vi "main.vi"() -> ()   [LabVIEW 2025]
uses:
  Module Main Cases.ctl
  71319344-41ff-4242-989e-c571bc358f37.vi
  <vilib>/Utility/error.llb/Clear Errors.vi
  <extravilib>/ChannelInstances/Event Messenger-c(str,var)/Instantiate.vi
  <extravilib>/ChannelInstances/Event Messenger-c(str,var)/))Channel.vi
  Channel Messages/9242 error converting cmd string to case enum--error.vi
  Channel Messages/Bundle Module Message/Bundle Module Message.xnode
  Module2/Module 2.lvlib
  Common-LabVIEW-Helpers/Source/Common Helpers.lvlib
  <extravilib>/ChannelInstances/Event Messenger-c(str,var).lvlib
panel:
  out "Sum Result":dbl
  in  "Sum":bool
  in  "Summand B":dbl
  in  "Summand A":dbl
  out "last ack data":cluster{"ident":string, "error":errorcluster}
  in  "module_interface":map{string, variant}(c390)={"Last Ack"=variant(cluster{"ident":string, "error":errorcluster} {"ident"="", "error"={"status"=FALSE, "code"=0, "source"=""}}), "Sum Result"=variant(dbl 0.0)}
  in  "Show Module2":bool
  in  "Show Module1":bool
  in  "Process Stop Button":bool
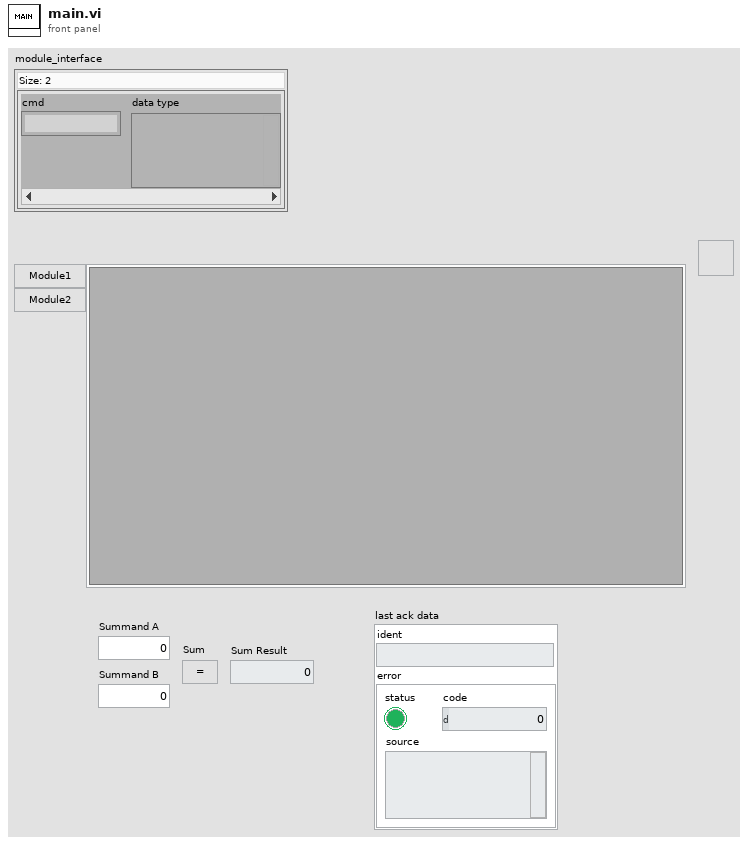
[diagram p1: front panel]
types:
  T1 = typedef "Module Main Cases.ctl" = enum16{"Last Ack", "Sum Result"}
  T2 = typedef "Event Messenger-c(str,var).lvlib/))Channel.ctl" = refnum<queue>
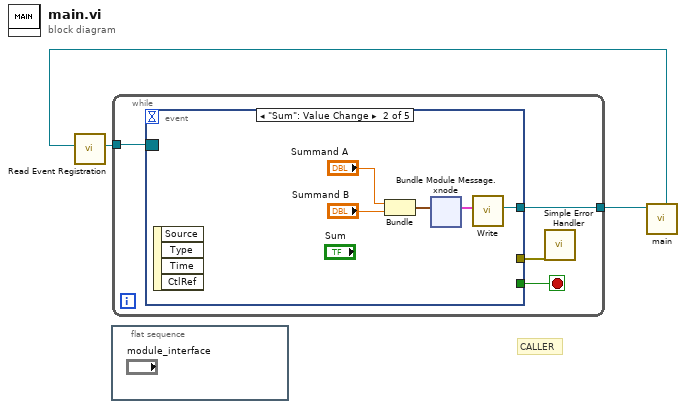
[diagram p0: block diagram]
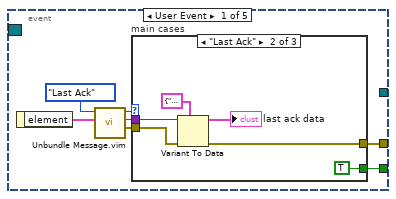
[diagram p2: hidden frame]
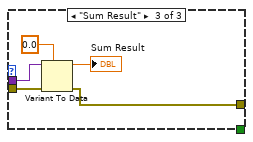
[diagram p4: hidden frame]
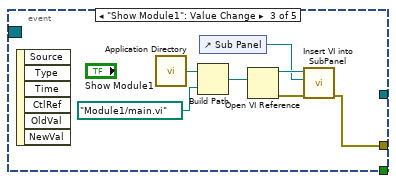
[diagram p5: hidden frame]
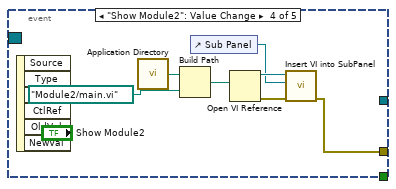
[diagram p6: hidden frame]
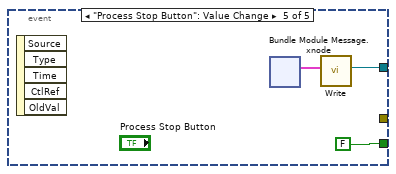
[diagram p7: hidden frame]
diagram:
  # "CALLER"
  n1 = flat-sequence {
    frame #0 {
    }
  }
  n2 = call <extravilib>:"Read Event Registration.vi"("channel"=w2) -> ("event registration refnum"=w1:refnum<event-registration>)  [unwired: 10 in]
  n3 = while {
    tunnel: [w6] -> w3
    tunnel: w1 -> [w4]
    stop <- w7 stop-if-true
    n4 = event shown="[1] \"Sum\": Value Change" {
      selector: w4 -> [_ _ _ _ _]
      dyn-events: _ -> [_ _ _ _ _]
      timeout: _ -> [_ _ _ _ _]
      tunnel: [w8 _ _ _ FALSE] -> w7
      tunnel: [_ w28 _ _ w51] -> w6
      tunnel: [w11 _ w37 w44 _] -> w5
      event User Event {
        n5 = event-data() -> ("element"=w9:cluster{"cmd":string, "data":variant})  [unwired: 1 in]
        n6 = call "Unbundle Message.vim"("message"=w9, "case type"=Module_Main_Cases."Last Ack" ("main cases")) -> ("error out"=w10:errorcluster, "data"=w12:variant, "case"=w13:T1)  [unwired: 7 in]
        n7 = case "main cases" shown="\"Last Ack\"" w13 {
          tunnel: w12 -> [_ w21 w25]
          tunnel: [w15 w20 w22] -> w11
          tunnel: w10 -> [w15 w19 w26]
          tunnel: [_ TRUE _] -> w8
          frame Default {
          }
          frame "Last Ack" {
            n8 = Variant To Data(error in=w19, type=cluster{"ident":string, "error":errorcluster} {"ident"="", "error"={"status"=FALSE, "code"=0, "source"=""}}, Variant=w21) -> (data=→"last ack data":cluster{"ident":string, "error":errorcluster}, error out=w20:errorcluster)
          }
          frame "Sum Result" {
            n9 = Variant To Data(error in=w26, type=0.0, Variant=w25) -> (data=→"Sum Result":dbl, error out=w22:errorcluster)
          }
        }
      }
      event "Sum": Value Change {
        n10 = event-data() -> ()  [unwired: 1 in, 4 out]
        n11 = Bundle("Summand A"="Summand A", "Summand B"="Summand B") -> (w27:cluster{"Summand A":dbl, "Summand B":dbl})  [unwired: 1 in]
        n12 = xnode "Bundle Module Message.xnode"("data"=w27) -> ("message"=w29:cluster{"cmd":string, "data":variant})  [unwired: 1 in, 1 out]
        n13 = call <extravilib>:"Write.vi"("element"=w29) -> ("channel"=w28:T2)  [unwired: 9 in, 1 out]
      }
      event "Show Module1": Value Change {
        n14 = event-data() -> ()  [unwired: 1 in, 6 out]
        n15 = call <vilib>:"Application Directory.vi"() -> ("Application Directory"=w43:path)
        n16 = Build Path(base path=w43, name or relative path=path "Module1/main.vi") -> (appended path=w42:path)
        n17 = control-ref of="Sub Panel"() -> (w39:refnum<vi>)
        n18 = Open VI Reference(vi path=w42) -> (vi reference=w41:refnum<vi>, error out=w40:errorcluster)  [unwired: 5 in]
        n19 = call "Insert VI into SubPanel.vi"("error in"=w40, "SubPnl Ref"=w39, "VI Ref"=w41) -> ("error out"=w37:errorcluster)  [unwired: 7 in, 1 out]
      }
      event "Show Module2": Value Change {
        n20 = event-data() -> ()  [unwired: 1 in, 6 out]
        n21 = call <vilib>:"Application Directory.vi"() -> ("Application Directory"=w50:path)
        n22 = Build Path(base path=w50, name or relative path=path "Module2/main.vi") -> (appended path=w49:path)
        n23 = control-ref of="Sub Panel"() -> (w46:refnum<vi>)
        n24 = Open VI Reference(vi path=w49) -> (vi reference=w48:refnum<vi>, error out=w45:errorcluster)  [unwired: 5 in]
        n25 = call "Insert VI into SubPanel.vi"("error in"=w45, "SubPnl Ref"=w46, "VI Ref"=w48) -> ("error out"=w44:errorcluster)  [unwired: 7 in, 1 out]
      }
      event "Process Stop Button": Value Change {
        n26 = event-data() -> ()  [unwired: 1 in, 5 out]
        n27 = xnode "Bundle Module Message.xnode"() -> ("message"=w52:cluster{"cmd":string, "data":variant})  [unwired: 2 in, 1 out]
        n28 = call <extravilib>:"Write.vi"("element"=w52) -> ("channel"=w51:T2)  [unwired: 9 in, 1 out]
      }
    }
    n29 = call <vilib>:"Simple Error Handler.vi"("error in (no error)"=w5) -> ()  [unwired: 4 in, 5 out]
  }
  n30 = call "main.vi"("Message In"=w3) -> ("Message Out"=w2:T2)  [unwired: 10 in]
